vi "select.vi"(3 "error in (no error)":errorcluster caption="错误输入（无错误）") -> (7 "out":T1, 10 "error out":errorcluster caption="错误输出")   [LabVIEW 2019]
uses:
  select.ctl
panel:
  in  "布尔":T1
  in  "?":bool
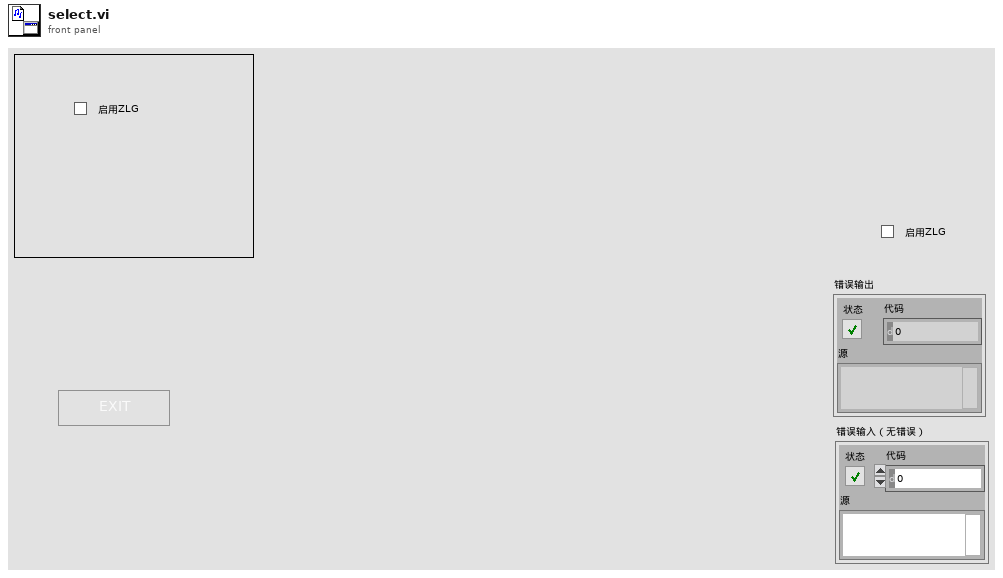
[diagram p1: front panel]
types:
  T1 = typedef "select.ctl" = bool
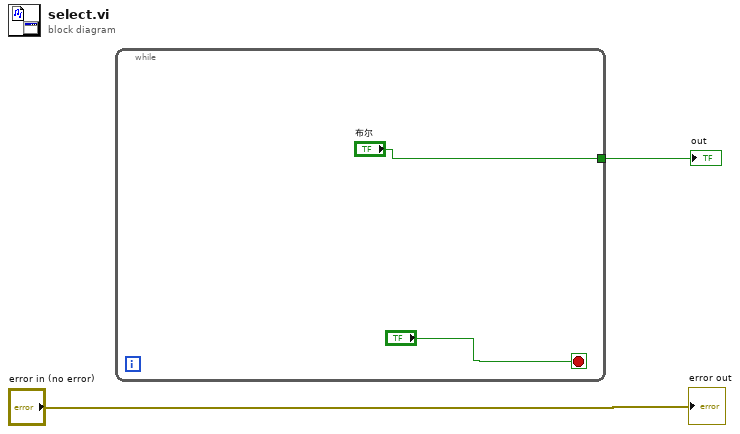
[diagram p0: block diagram]
diagram:
  n1 = while {
    tunnel: ["布尔"] -> w1
    stop <- "?" stop-if-true
  }
  "out" <- w1
  "error out" <- "error in (no error)"
